vi "checkChannelsCreated.vi"(8 "error in (no error)":errorcluster, 11 "Connection.LocalQueue in":refnum<class "Connection.LocalQueue.lvclass">) -> (0 "error out":errorcluster, 1 "outbound created":bool, 2 "inbound created":bool, 3 "Connection.LocalQueue out":refnum<class "Connection.LocalQueue.lvclass">)   [LabVIEW 2013, in "Connection.Queue_GOSPL.lvlib" / "Connection.LocalQueue.lvclass"]
uses:
  Connection.LocalQueue.lvclass
  Connection/Connection.lvclass
  Connection.LocalQueue.lvclass/Connection.LocalQueue.ctl
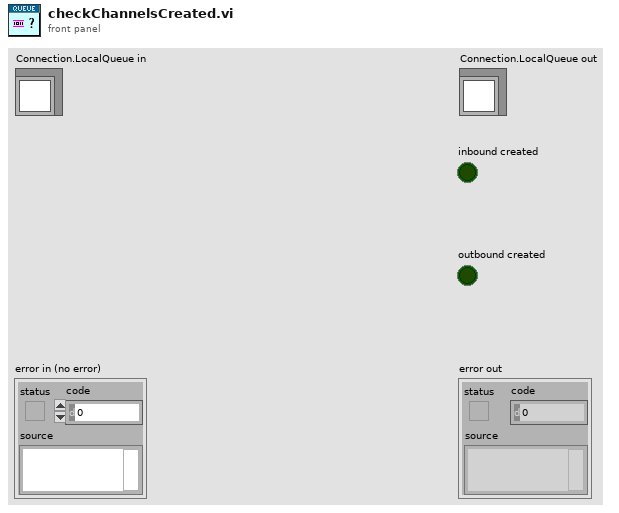
[diagram p1: front panel]
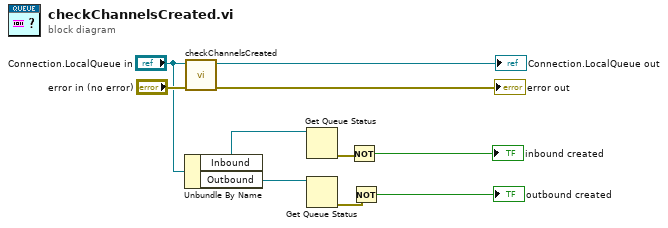
[diagram p0: block diagram]
diagram:
  n1 = Unbundle By Name("Connection.LocalQueue in") -> ("Inbound"=w6:refnum<queue>, "Outbound"=w5:refnum<queue>)
  n2 = call-parent "checkChannelsCreated.vi"("error in (no error)"="error in (no error)", "Connection in"="Connection.LocalQueue in") -> ("error out"=→"error out":errorcluster, "Connection out"=→"Connection.LocalQueue out":refnum<class "Connection.LocalQueue.lvclass">)  [unwired: 6 in, 2 out]
  n3 = Get Queue Status(queue=w6) -> (error out=w4:errorcluster)  [unwired: 2 in, 7 out]
  n4 = Get Queue Status(queue=w5) -> (error out=w3:errorcluster)  [unwired: 2 in, 7 out]
  n5 = Not(x=w4) -> (.not. x?=→"inbound created":bool)
  n6 = Not(x=w3) -> (.not. x?=→"outbound created":bool)
